vi "ReteachTravPosition.vi"(3 "Mode":T1, 5 "Traverse line In":T2 {"Carrier_2 Q (l/min)" format="%#.2f"; "Row Duration (mins)" format="%#.1f"; "Row No" min=0; "Trace Gas Concentration (%)" min=0.0 format="%#_4f"; "Carrier_1 Q (l/min)" format="%#.4f"; "Tunnel Speed" format="%#.2f"; "Start X" format="%#.2f"; "Start Y" format="%#.2f"; "Start Z" format="%#.2f"; "End X" format="%#.2f"; "End Y" format="%#.2f"; "End Z" format="%#.2f"; "Averaging time (min)" min=0.0 format="%#.2f"}) -> (0 "Error Message":string, 1 "Status":T5, 2 "Traverse line Out":T2 {"Carrier_2 Q (l/min)" format="%#.2f"; "Row Duration (mins)" format="%#.1f"; "Row No" min=0; "Trace Gas Concentration (%)" min=0.0 format="%#_4f"; "Carrier_1 Q (l/min)" format="%#.4f"; "Tunnel Speed" format="%#.2f"; "Start X" format="%#.2f"; "Start Y" format="%#.2f"; "Start Z" format="%#.2f"; "End X" format="%#.2f"; "End Y" format="%#.2f"; "End Z" format="%#.2f"; "Averaging time (min)" min=0.0 format="%#.2f"})   [LabVIEW 2020]
uses:
  Gen Trav/Multi_Run_Status.ctl
  Gen Trav/Trav_mode.ctl
  Controls/Home.ctl
  Gen Trav/Spacing.ctl
  Controls/Multi_run_mode.ctl
  Gen Trav/Traverse_cluster.ctl
  Controls/User_Specific_mode.ctl
panel:
  out "Model  Roll        Pitch       Yaw (deg)":sgl[](array[numeric]) format="%#.2f"
  in  "Traverse Name":string
  # "X           Y            Z"
  # "Start"
  # "End"
  # "X           Y            Z"
  # "Start"
  # "End"
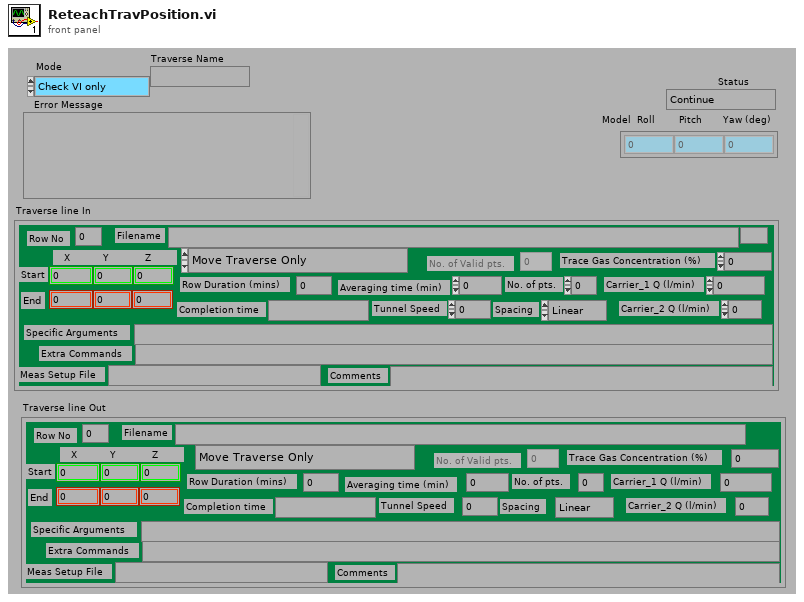
[diagram p1: front panel]
types:
  T1 = typedef "User_Specific_mode.ctl" = enum16{"Check VI only", "Run VI"}
  T2 = typedef "Traverse_cluster.ctl" = cluster{"Start X":sgl, "Start Y":sgl, "Start Z":sgl, "End X":sgl, "End Y":sgl, "End Z":sgl, "No. of pts.":i32, "Spacing":T3, "Filename":path, "Tunnel Speed":dbl, "Averaging time (min)":dbl, "Extra Commands":string, "Carrier_1 Q (l/min)":dbl, "Carrier_2 Q (l/min)":dbl, "Trace Gas Concentration (%)":dbl, "Specific Arguments":string, "Comments":string, "Row No":i32, "Row Type Selector":T4, "Completion time":string, "Row Duration (mins)":dbl, "No. of Valid pts.":i32, "Meas Setup File":string}
  T3 = typedef "Spacing.ctl" = enum16{"Linear", "Log", "Gauss", "Specified", "N/A"}
  T4 = typedef "Multi_run_mode.ctl" = enum16{"Move Traverse Only", "Set Tunnel Speed Only", "Set Source Only", "Set Measurement Conditions", "Single Measurement", "Vertical Profile", "Lateral Profile", "Longitudinal Profile", "Multi-Axis Profile", "Explore Volume", "Auto Calibrate", "Meas Fast FID Bkgnd", "Check Beam Power", "Scanning Valve Measurement", "Run VI Named:", "Set ADAM Ch", "Wait (minutes)", "Send Message", "Synchronize With:", "Fall Back to this Row", "Turn Off Row Repeating", "Traverse 3D Volume", "Blank Row", "Jump to Fall Back Row"}
  T5 = typedef "Multi_Run_Status.ctl" = enum16{"Continue", "Continue with Error", "Jump to Next Point", "Jump to Next Row", "Jump To Fall Back", "Terminate Run"}
  T6 = typedef "Trav_mode.ctl" = enum16{"Move traverse", "Read traverse position", "Teach Position"}
  T7 = enum16{"To Traverse Coordinates", "To User Coordinates"}
  T8 = typedef "Home.ctl" = enum16{"Don't Home", "Home  +X", "Home  -X", "Home  +Y", "Home  -Y", "Home  +Z", "Home  -Z"}
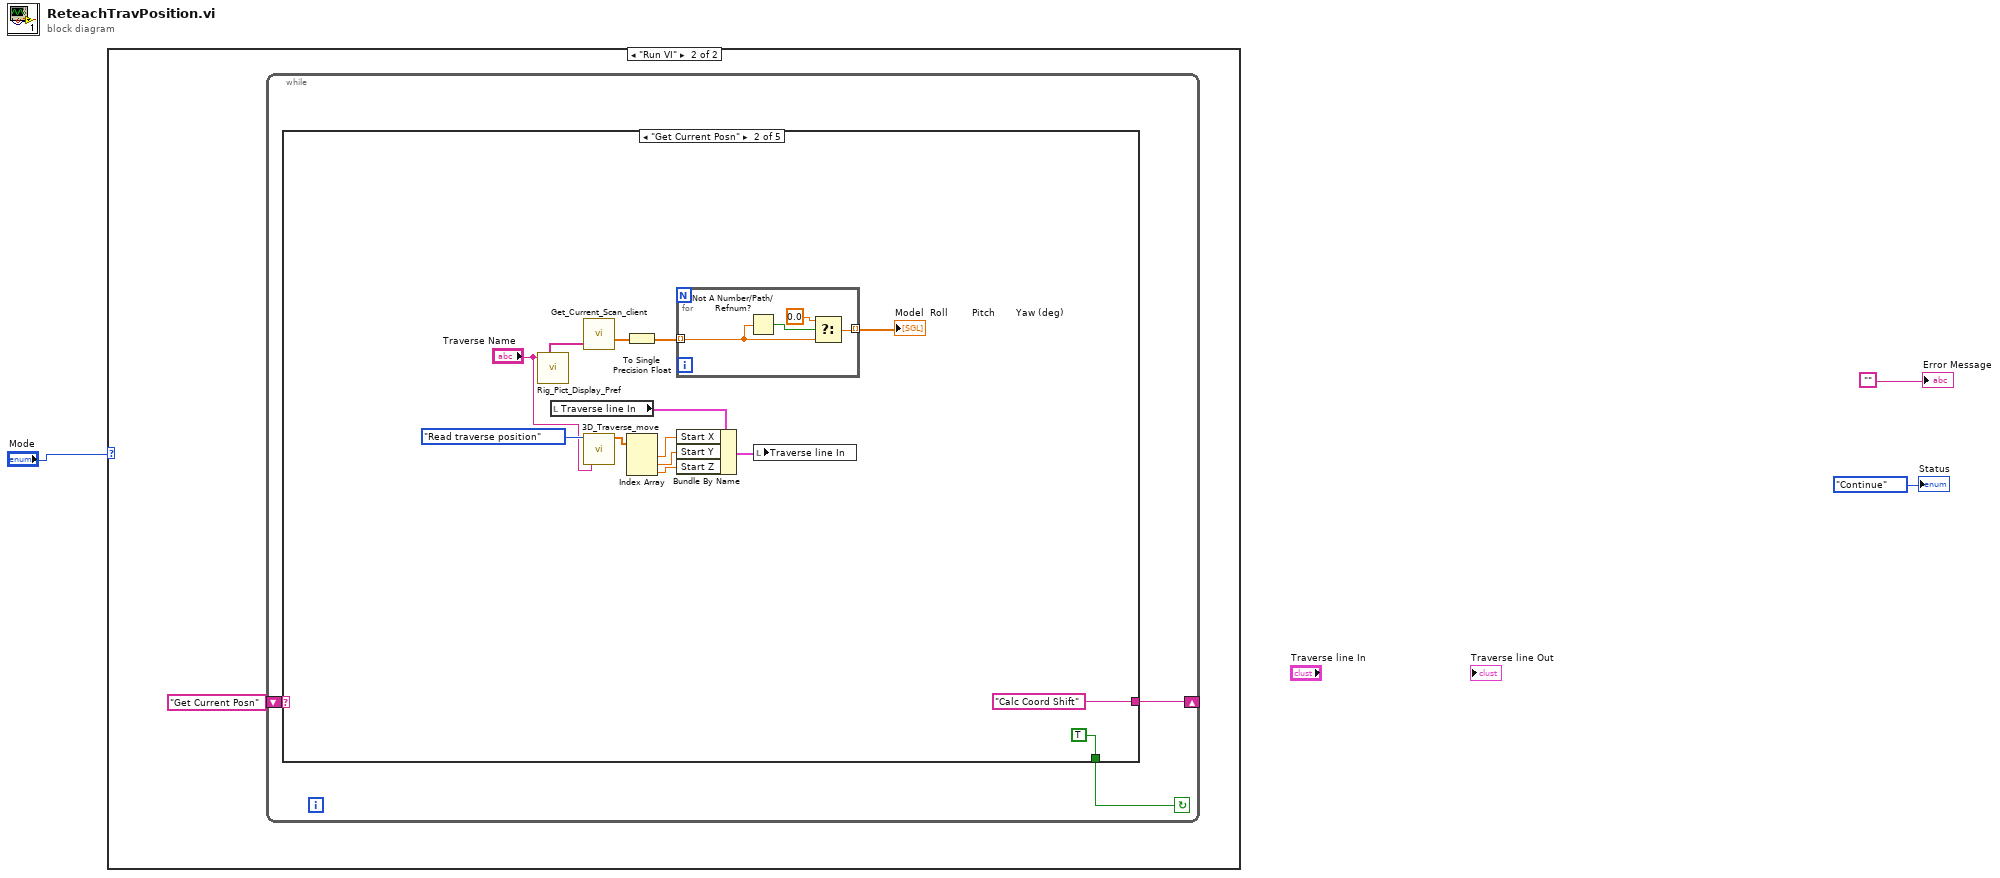
[diagram p0: block diagram]
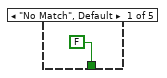
[diagram p3: hidden frame]
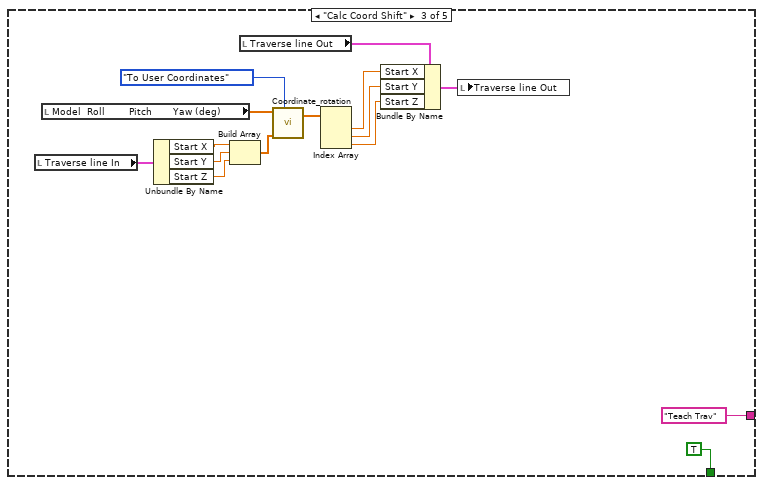
[diagram p4: hidden frame]
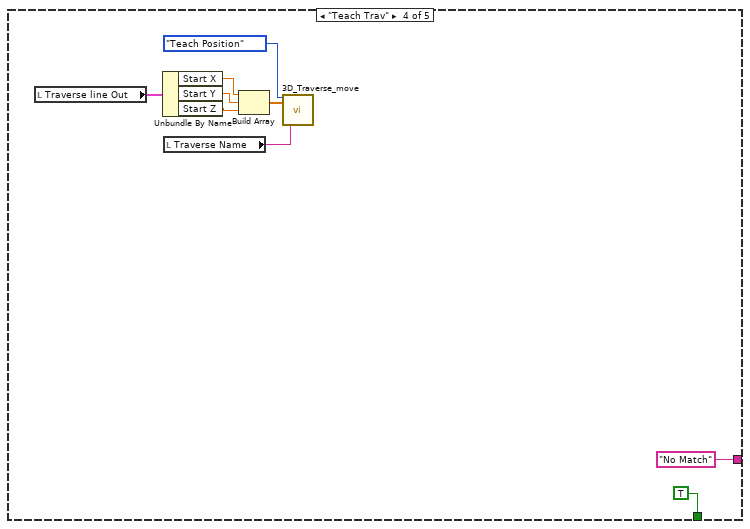
[diagram p5: hidden frame]
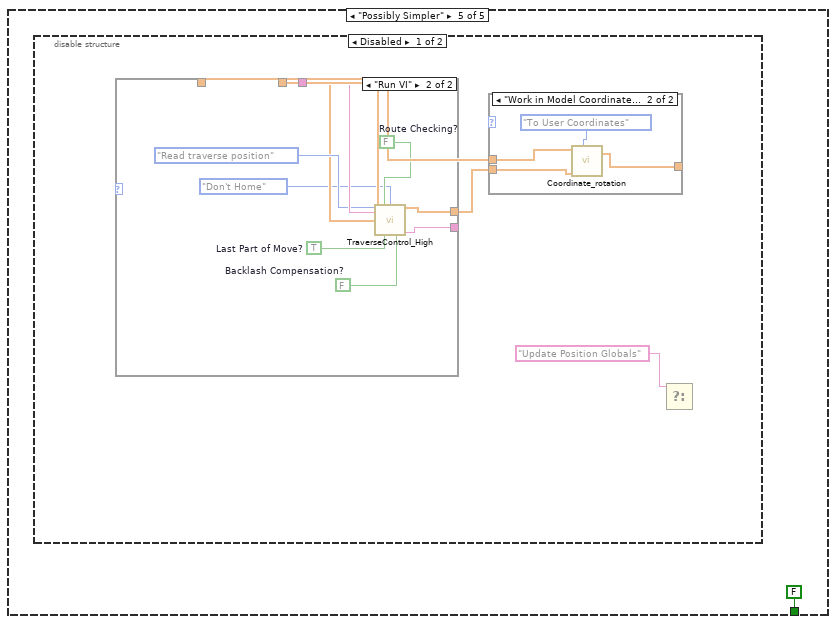
[diagram p6: hidden frame]
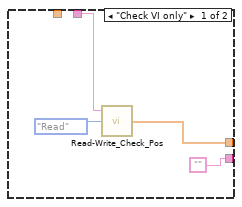
[diagram p7: hidden frame]
diagram:
  n1 = case shown="\"Run VI\"" "Mode" {
    frame "Check VI only", Default {
    }
    frame "Run VI" {
      n2 = while {
        shift-right: [w6] -> _
        shift-left: "Get Current Posn" -> [w7]
        stop <- w5 continue-if-true
        n3 = case shown="\"Get Current Posn\"" w7 {
          tunnel: [_ "Calc Coord Shift" "Teach Trav" "No Match" _] -> w6
          tunnel: [FALSE TRUE TRUE TRUE FALSE] -> w5
          frame "No Match", Default {
          }
          frame "Get Current Posn" {
            n4 = call "Rig_Pict_Display_Pref.vi"("Traverse Name"="Traverse Name") -> ("Roll Pitch Yaw ADAM Channels"=w14:string[])  [unwired: 3 in, 4 out]
            n5 = local read "Traverse line In"() -> (w19:T2)
            n6 = call "Get_Current_Scan_client.vi"("multipleChannels"=w14) -> ("Numerical Values"=w13:dbl[])  [unwired: 2 in, 2 out]
            n7 = call "3D_Traverse_move.vi"("Mode"=Trav_mode."Read traverse position", "Traverse name"="Traverse Name") -> ("Trav Position achieved"=w18:sgl[])  [unwired: 14 in, 3 out]
            n8 = To Single Precision Float(number=w13) -> (single precision float=w12:sgl[])
            n9 = Index Array(array=w18) -> (element #1=w17:sgl, element #2=w16:sgl, element #3=w15:sgl)  [unwired: 3 in]
            n10 = for {
              tunnel: w12 -> [w25] mode=indexing
              tunnel: [w23] -> w11 mode=indexing
              n11 = Not A Number/Path/Refnum?(number/path/refnum=w25) -> (NaN/Path/Refnum?=w26:bool)
              n12 = Select(t=sgl 0.0, s=w26, f=w25) -> (s? t:f=w23:sgl)
            }
            "Model  Roll        Pitch       Yaw (deg)" <- w11
            n13 = Bundle By Name(cluster=w19, "Start X"=w17, "Start Y"=w16, "Start Z"=w15) -> (w10:T2)
            n14 = local write "Traverse line In"(w10) -> ()
          }
          frame "Calc Coord Shift" {
            n15 = local read "Traverse line In"() -> (w37:T2)
            n16 = local read "Model  Roll        Pitch       Yaw (deg)"() -> (w39:sgl[])
            n17 = Unbundle By Name(w37) -> ("Start X"=w36:sgl, "Start Y"=w35:sgl, "Start Z"=w34:sgl)
            n18 = Build Array(w36, w35, w34) -> (w33:sgl[])
            n19 = local read "Traverse line Out"() -> (w32:T2)
            n20 = call "Coordinate_rotation.vi"("Roll-Pitch-Yaw"=w39, "Input Position"=w33, "Mode"=T7."To User Coordinates") -> ("Output Position"=w31:sgl[])  [unwired: 2 in, 1 out]
            n21 = Index Array(array=w31) -> (element #1=w30:sgl, element #2=w29:sgl, element #3=w28:sgl)  [unwired: 3 in]
            n22 = Bundle By Name(cluster=w32, "Start X"=w30, "Start Y"=w29, "Start Z"=w28) -> (w27:T2)
            n23 = local write "Traverse line Out"(w27) -> ()
          }
          frame "Teach Trav" {
            n24 = local read "Traverse line Out"() -> (w47:T2)
            n25 = Unbundle By Name(w47) -> ("Start X"=w46:sgl, "Start Y"=w45:sgl, "Start Z"=w44:sgl)
            n26 = local read "Traverse Name"() -> (w42:string)
            n27 = Build Array(w46, w45, w44) -> (w43:sgl[])
            n28 = call "3D_Traverse_move.vi"("Mode"=Trav_mode."Teach Position", "Position"=w43, "Traverse name"=w42) -> ()  [unwired: 13 in, 4 out]
          }
          frame "Possibly Simpler" {
            n29 = disable-structure shown="Disabled" {
              frame Disabled {
                n30 = Select(t="Update Position Globals") -> ()  [unwired: 2 in, 1 out]
                n31 = case shown="\"Run VI\"" {
                  selector: _ -> [_ _]
                  tunnel: _ -> [w57 w68]
                  tunnel: ["" w70] -> w56
                  tunnel: w54 -> [_ w64]
                  tunnel: [w58 w69] -> w53
                  tunnel: _ -> [_ w63]
                  frame "Check VI only" {
                    n32 = call "Read-Write_Check_Pos.vi"("Mode"=enum16{"Read", "Write"}."Read", "Traverse Name"=w57) -> ("Position Output"=w58:sgl[])  [unwired: 1 in]
                  }
                  frame "Run VI" {
                    w62 = TRUE  # Last Part of Move?
                    w67 = FALSE  # Route Checking?
                    w66 = FALSE  # Backlash Compensation?
                    n33 = call "TraverseControl_High.vi"("Mode"=Trav_mode."Read traverse position", "Route Checking?"=w67, "Home"=Home."Don't Home", "Traverse Name"=w68, "Model       Roll      Pitch       Yaw (deg)"=w64, "Position input XYZ Always Tunnel"=w63, "Last Part of Move?"=w62, "Backlash Compensation?"=w66) -> ("Position Output XYZ"=w69:sgl[], "Error String"=w70:string)  [unwired: 6 in]
                  }
                }
                n34 = case shown="\"Work in Model Coordinates\"" w55 {
                  tunnel: w53 -> [w71 w73]
                  tunnel: [w71 w74] -> _
                  tunnel: [_ w72] -> w54
                  frame "Work in Tunnel Coordinates" {
                  }
                  frame "Work in Model Coordinates" {
                    n35 = call "Coordinate_rotation.vi"("Roll-Pitch-Yaw"=w72, "Input Position"=w73, "Mode"=T7."To User Coordinates") -> ("Output Position"=w74:sgl[])  [unwired: 2 in, 1 out]
                  }
                }
              }
              frame Enabled {
              }
            }
          }
        }
      }
    }
  }
  "Status" <- Multi_Run_Status."Continue" ("Status")
  "Error Message" <- "" ("Error Message")
